vi "Timer.vi"(1 "key":T2(ring), 2 "t2":u32, 3 "t1":u32) -> (0 "Timings":dbl[][](array[numeric])=[[2417234066.0, 52858.0]] format="%^#_4g")   [LabVIEW 2013]
panel:
  out "ADC wait/meas loop":dbl
  in  "key list":T1(array[ring])=[enum."total time", enum."read config", enum."plot loop", enum."save data", enum."config instr", enum."FPGA config", enum."voltmeter init", enum."initial move", enum."read init val", enum."meas loop", enum."move", enum."step wait", enum."FPGA reset", enum."FPGA start", enum."read data", enum."FPGA stop", enum."clear buffer", enum."ADC wait", enum."ADC get", enum."ADC treat"]
  out "read/meas loop":dbl
  out "read/total":dbl
  # "total (s)"
  # "average (ms)"
  # "min (ms)"
  # "max (ms)"
  # "nb of calls"
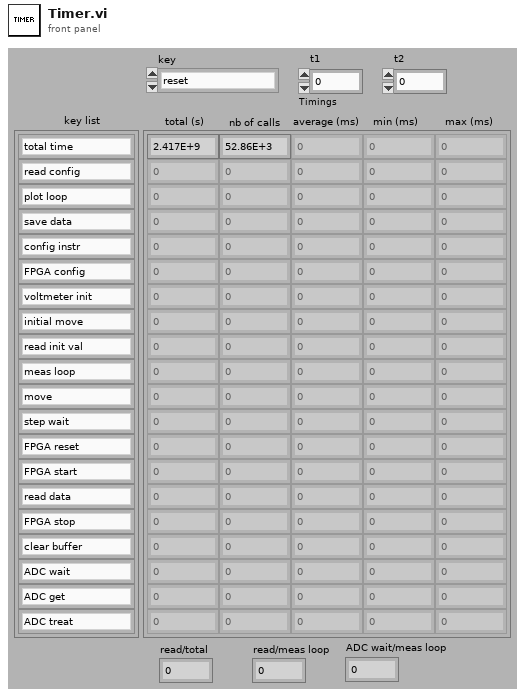
[diagram p1: front panel]
types:
  T1 = enum16{"reset", "total time", "read config", "plot loop", "save data", "config instr", "FPGA config", "voltmeter init", "initial move", "read init val", "meas loop", "move", "step wait", "FPGA reset", "FPGA start", "read data", "FPGA stop", "clear buffer", "ADC wait", "ADC get", "ADC treat"}[]
  T2 = enum16{"reset", "total time", "read config", "plot loop", "save data", "config instr", "FPGA config", "voltmeter init", "initial move", "read init val", "meas loop", "move", "step wait", "FPGA reset", "FPGA start", "read data", "FPGA stop", "clear buffer", "ADC wait", "ADC get", "ADC treat"}
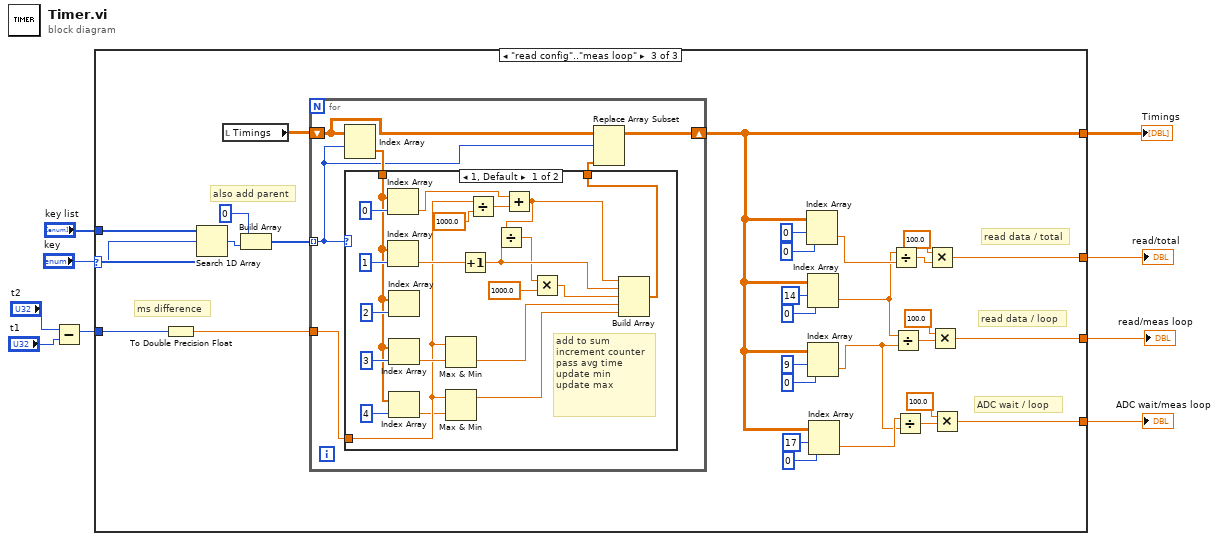
[diagram p0: block diagram]
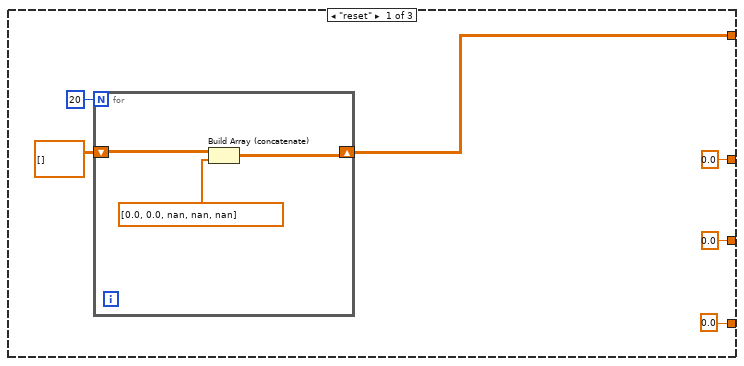
[diagram p2: hidden frame]
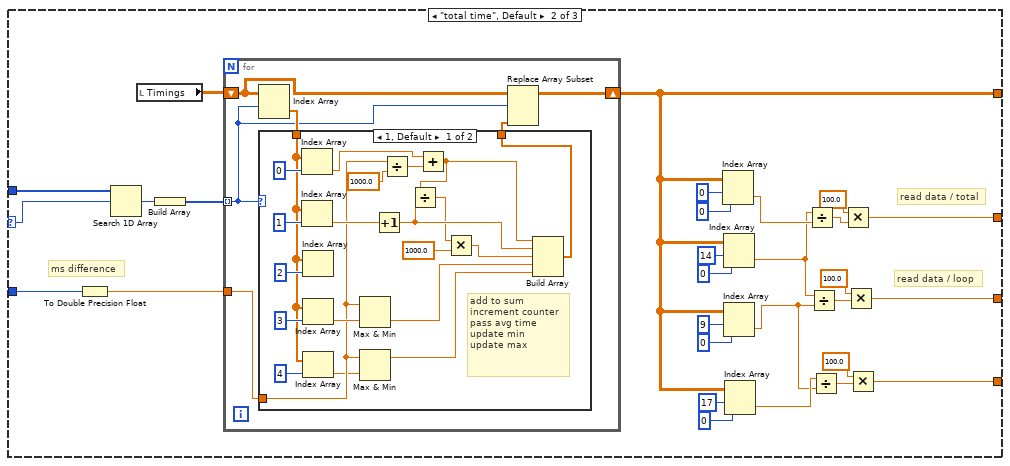
[diagram p3: hidden frame]
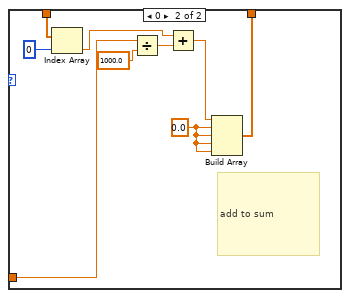
[diagram p4: hidden frame]
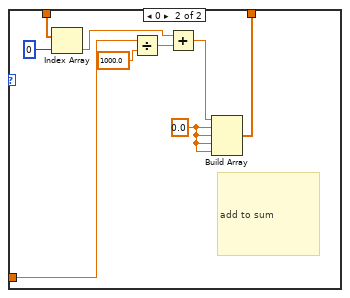
[diagram p5: hidden frame]
diagram:
  n1 = Subtract(x="t2", y="t1") -> (x-y=w5:u32)
  n2 = case shown="\"read config\"..\"meas loop\"" "key" {
    selector: "key" -> [_ w46 w112]
    tunnel: "key list" -> [_ w47 w113]
    tunnel: [w11 w21 w87] -> w4
    tunnel: [0.0 w31 w86] -> w3
    tunnel: [0.0 w30 w85] -> w2
    tunnel: w5 -> [_ w28 w108]
    tunnel: [0.0 w24 w84] -> w1
    frame "reset" {
      n3 = for {
        N: 20 -> [_]
        shift-right: [w17] -> w11
        shift-left: dbl[][] [] -> [w18]
        n4 = Build Array (concatenate)(w18, dbl[] [0.0, 0.0, nan, nan, nan]) -> (w17:dbl[][])
      }
    }
    frame "total time", Default {
      # "ms difference"
      # "read data / loop"
      # "read data / total"
      n5 = To Double Precision Float(number=w28) -> (double precision float=w27:dbl)
      n6 = Search 1D Array(1D array=w47, element=w46) -> (index of element=w45:i32)  [unwired: 1 in]
      n7 = local read "Timings"() -> (w44:dbl[][])
      n8 = Build Array(w45) -> (w29:i32[])
      n9 = for {
        shift-right: [w53] -> w21
        shift-left: w44 -> [w52]
        tunnel: w29 -> [w49] mode=indexing
        tunnel: w27 -> [w48]
        n10 = Index Array(array=w52, index (row)=w49) -> (element=w50:dbl[])  [unwired: 1 in]
        n11 = case shown="1, Default" w49 {
          tunnel: [w74 w83] -> w51
          tunnel: w50 -> [w64 w78]
          tunnel: w48 -> [w61 w77]
          frame 1, Default {
            # "add to sum\nincrement counter\npass avg time\nupdate min\nupdate max"
            n12 = Index Array(array=w64, index=0) -> (element=w70:dbl)
            n13 = Index Array(array=w64, index=1) -> (element=w68:dbl)
            n14 = Index Array(array=w64, index=2) -> ()  [unwired: 1 out]
            n15 = Index Array(array=w64, index=3) -> (element=w63:dbl)
            n16 = Index Array(array=w64, index=4) -> (element=w60:dbl)
            n17 = Max & Min(x=w61, y=w63) -> (min(x,y)=w62:dbl)  [unwired: 1 out]
            n18 = Max & Min(x=w61, y=w60) -> (max(x,y)=w59:dbl)  [unwired: 1 out]
            n19 = Increment(x=w68) -> (x+1=w57:dbl)
            n20 = Divide(x=w61, y=1000.0) -> (x/y=w73:dbl)
            n21 = Add(x=w70, y=w73) -> (x+y=w58:dbl)
            n22 = Divide(x=w58, y=w57) -> (x/y=w56:dbl)
            n23 = Multiply(x=w56, y=1000.0) -> (x*y=w54:dbl)
            n24 = Build Array(w58, w57, w54, w62, w59) -> (w74:dbl[])
          }
          frame 0 {
            w75 = 0.0 ("element")
            # "add to sum"
            n25 = Index Array(array=w78, index=0) -> (element=w79:dbl)
            n26 = Divide(x=w77, y=1000.0) -> (x/y=w82:dbl)
            n27 = Add(x=w79, y=w82) -> (x+y=w76:dbl)
            n28 = Build Array(w76, w75, w75, w75, w75) -> (w83:dbl[])
          }
        }
        n29 = Replace Array Subset(array=w52, new element=w51, index (row)=w49) -> (w53:dbl[][])  [unwired: 1 in]
      }
      n30 = Index Array(array=w21, index (row)=0, index (col)=0) -> (element=w39:dbl)
      n31 = Index Array(array=w21, index (row)=14, index (col)=0) -> (element=w38:dbl)
      n32 = Index Array(array=w21, index (row)=9, index (col)=0) -> (element=w19:dbl)
      n33 = Index Array(array=w21, index (row)=17, index (col)=0) -> (element=w20:dbl)
      n34 = Divide(x=w38, y=w39) -> (x/y=w40:dbl)
      n35 = Divide(x=w38, y=w19) -> (x/y=w42:dbl)
      n36 = Divide(x=w20, y=w19) -> (x/y=w25:dbl)
      n37 = Multiply(x=100.0, y=w40) -> (x*y=w31:dbl)
      n38 = Multiply(x=100.0, y=w42) -> (x*y=w30:dbl)
      n39 = Multiply(x=100.0, y=w25) -> (x*y=w24:dbl)
    }
    frame "read config".."meas loop" {
      # "ADC wait / loop"
      # "read data / loop"
      # "read data / total"
      # "also add parent"
      # "ms difference"
      n40 = To Double Precision Float(number=w108) -> (double precision float=w107:dbl)
      n41 = Search 1D Array(1D array=w113, element=w112) -> (index of element=w111:i32)  [unwired: 1 in]
      n42 = local read "Timings"() -> (w110:dbl[][])
      n43 = Build Array(0 ("element"), w111) -> (w109:i32[])
      n44 = for {
        shift-right: [w119] -> w87
        shift-left: w110 -> [w118]
        tunnel: w109 -> [w115] mode=indexing
        tunnel: w107 -> [w114]
        n45 = Index Array(array=w118, index (row)=w115) -> (element=w116:dbl[])  [unwired: 1 in]
        n46 = case shown="1, Default" w115 {
          tunnel: [w140 w149] -> w117
          tunnel: w116 -> [w130 w144]
          tunnel: w114 -> [w127 w143]
          frame 1, Default {
            # "add to sum\nincrement counter\npass avg time\nupdate min\nupdate max"
            n47 = Index Array(array=w130, index=0) -> (element=w136:dbl)
            n48 = Index Array(array=w130, index=1) -> (element=w134:dbl)
            n49 = Index Array(array=w130, index=2) -> ()  [unwired: 1 out]
            n50 = Index Array(array=w130, index=3) -> (element=w129:dbl)
            n51 = Index Array(array=w130, index=4) -> (element=w126:dbl)
            n52 = Max & Min(x=w127, y=w129) -> (min(x,y)=w128:dbl)  [unwired: 1 out]
            n53 = Max & Min(x=w127, y=w126) -> (max(x,y)=w125:dbl)  [unwired: 1 out]
            n54 = Increment(x=w134) -> (x+1=w123:dbl)
            n55 = Divide(x=w127, y=1000.0) -> (x/y=w139:dbl)
            n56 = Add(x=w136, y=w139) -> (x+y=w124:dbl)
            n57 = Divide(x=w124, y=w123) -> (x/y=w122:dbl)
            n58 = Multiply(x=w122, y=1000.0) -> (x*y=w120:dbl)
            n59 = Build Array(w124, w123, w120, w128, w125) -> (w140:dbl[])
          }
          frame 0 {
            w141 = 0.0 ("element")
            # "add to sum"
            n60 = Index Array(array=w144, index=0) -> (element=w145:dbl)
            n61 = Divide(x=w143, y=1000.0) -> (x/y=w148:dbl)
            n62 = Add(x=w145, y=w148) -> (x+y=w142:dbl)
            n63 = Build Array(w142, w141, w141, w141, w141) -> (w149:dbl[])
          }
        }
        n64 = Replace Array Subset(array=w118, new element=w117, index (row)=w115) -> (w119:dbl[][])  [unwired: 1 in]
      }
      n65 = Index Array(array=w87, index (row)=0, index (col)=0) -> (element=w101:dbl)
      n66 = Index Array(array=w87, index (row)=14, index (col)=0) -> (element=w100:dbl)
      n67 = Index Array(array=w87, index (row)=9, index (col)=0) -> (element=w88:dbl)
      n68 = Index Array(array=w87, index (row)=17, index (col)=0) -> (element=w89:dbl)
      n69 = Divide(x=w100, y=w101) -> (x/y=w102:dbl)
      n70 = Divide(x=w100, y=w88) -> (x/y=w104:dbl)
      n71 = Divide(x=w89, y=w88) -> (x/y=w92:dbl)
      n72 = Multiply(x=100.0, y=w102) -> (x*y=w86:dbl)
      n73 = Multiply(x=100.0, y=w104) -> (x*y=w85:dbl)
      n74 = Multiply(x=100.0, y=w92) -> (x*y=w84:dbl)
    }
  }
  "Timings" <- w4
  "read/total" <- w3
  "read/meas loop" <- w2
  "ADC wait/meas loop" <- w1
